vi "Read Dataset.vi"(8 "error in":errorcluster, 11 "Network Stream in":refnum<class "Network Stream.lvclass">) -> (0 "error out":errorcluster, 3 "Network Stream out":refnum<class "Network Stream.lvclass">)   [LabVIEW 2019, in "Network Stream.lvlib" / "Network Stream.lvclass"]
uses:
  Network Stream.lvclass
  C:/Program Files (x86)/National Instruments/LabVIEW 2019/vi.lib/ActorFramework/Actor/Actor.lvclass
  <vilib>/ActorFramework/Actor/Actor.lvclass/Actor.ctl
  Network Stream.lvclass/Network Stream.ctl
  Network Stream Messages/Dataset Msg/Dataset Msg.lvclass/Dataset Msg.ctl
  <vilib>/ActorFramework/Message Enqueuer/Message Enqueuer.lvclass/Message Enqueuer.ctl
  Network Stream Messages/NS Connection Msg/NS Connection Msg.lvclass/NS Connection Msg.ctl
  <vilib>/ActorFramework/Message Enqueuer/Enqueue.vi
  Network Stream Messages/Dataset Msg/Dataset Msg.lvclass
  C:/Program Files (x86)/National Instruments/LabVIEW 2019/vi.lib/ActorFramework/Message/Message.lvclass
  Network Stream Messages/NS Connection Msg/NS Connection Msg.lvclass
  <vilib>/ActorFramework/Message Priority Queue/Priority Enqueue.vi
  <resource>/objmgr/ni.dex.rc
  <vilib>/ActorFramework/Actor/Actor.lvclass
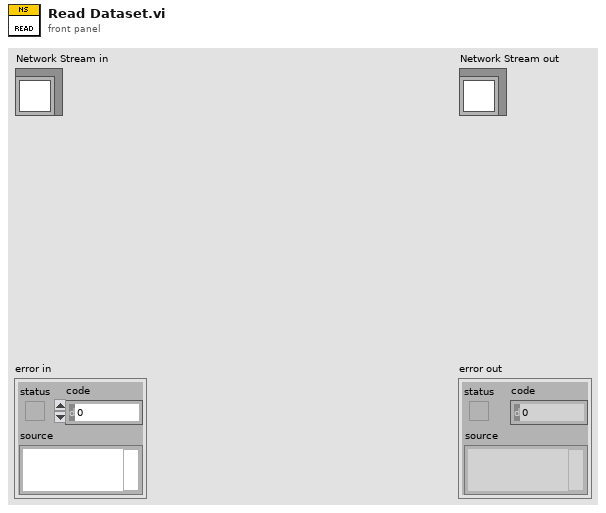
[diagram p1: front panel]
types:
  T1 = cluster{"System Status":cluster{"Power On Off":bool, "Discharge Temp":dbl, "Liquid Temp":dbl, "Suction Temp":dbl, "Ambient Temp":dbl, "Sleep":bool, "System Status":u16, "M1 Actuated":bool, "M2 Actuated":bool, "Sleep Timer":dbl, "M1 Bin":cluster{"Bin String":string, "Bin Color":u16}, "M2 Bin":cluster{"Bin String":string, "Bin Color":u16}, "Discharge Pressure":dbl, "Suction Pressure":dbl, "Compression Ratio":dbl, "Compressor Amps":dbl, "Compressor Hours":dbl, "Bypass Steps":u16, "SubCooling":dbl, "SuperHeat":dbl, "Serial Number":string, "EMO detected":bool, "EMO Tripped":bool, "Thermal cutoff":bool, "Thermal cutoff 2":bool, "High Pressure switch":bool, "Running Time":timestamp, "SOM Status":cluster{"Boot Up Time":timestamp, "Software Version":string, "CPU Usage":dbl, "Memory Available":dbl, "SD card free space":dbl, "SOM Storage":dbl}, "Cascade Extra":cluster{"Discharge Temp High Side":dbl, "Suction Temp High Side":dbl, "Liquid Temp High side":dbl, "Discharge Pressure 2":dbl, "Suction Pressure 2":dbl, "Low Side RPM":dbl, "High Side RPM":dbl}}, "M1 Status":cluster{"Case Temp":dbl, "Evap Temp":dbl, "Heater %":dbl, "EEV Steps":u32, "Set Temp":dbl, "Feedback":u8, "Power Drive":bool, "Piston Volts":dbl, "Safe Temp":bool, "Power":bool, "Thermal State":u16, "Error":bool, "In tollerance":bool, "Head State":u16, "Piston Force":dbl, "Package":string, "Dynamic SV":dbl, "PV":dbl, "TSD Temp":dbl, "DC Load Watts":dbl, "AC Load Watts":dbl, "Intec Feedback":dbl}, "M2 Status":cluster{"Case Temp":dbl, "Evap Temp":dbl, "Heater %":dbl, "EEV Steps":u32, "Set Temp":dbl, "Feedback":u8, "Power Drive":bool, "Piston Volts":dbl, "Safe Temp":bool, "Power":bool, "Thermal State":u16, "Error":bool, "In tollerance":bool, "Head State":u16, "Piston Force":dbl, "Package":string, "Dynamic SV":dbl, "PV":dbl, "TSD Temp":dbl, "DC Load Watts":dbl, "AC Load Watts":dbl, "Intec Feedback":dbl}, "Config Data":cluster{"Packages":cluster{"DUT Force lbf":cluster{" 0":u32, " 1":u32, " 2":u32, "3":u32, "4":u32, "5":u32, " 6":u32, "7":u32, "8":u32, "9":u32}, "DUT Names":cluster{"0":string, "1":string, "2":string, "3":string, "4":string, "5":string, "6":string, "7":string, "8":string, "9":string}}, "Heater PID":cluster{"P":dbl, "I":dbl, "D":dbl}, "Piston Settings":cluster{"Forces Slope":dbl, "Forces Intercept":dbl, "Transition Force":dbl, "Up Force":dbl, "Diameter (mm)":dbl, "Delay (ms)":dbl, "Pressure Ramp Delay (ms)":dbl}, "Safe Temps":cluster{"Minimum":i32, "Enabled":bool, "Maximum":i32}, "System Settings":cluster{"Number of Heads":i32, "60Hz Power":bool, "FTC200":bool, "AutoStartup":bool, "Purge":bool, "Sensors":bool, "HandClamp":bool, "ATE":bool, "Benchtop":bool, "Production":bool, "Refrigerant":u16, "Handler":bool, "Shuttle":bool, "220V":bool, "Cascade":bool, "Suction Sensor":u16, "Discharge Sensor":u16}, "Stepper Settings ":cluster{"Microstepping":u16, "Velocity":u8}, "Set Point Range":cluster{"Max":dbl, "Min":dbl}, "Pedestal Check DeltaT":dbl, "Ramp Delta T":dbl, "Ramp-SS Threshold":dbl, "SS Tolerance":dbl, "EEV PID":cluster{"Ramp Up Target":dbl, "Ramp Down Target":dbl, "Steady State Target":dbl, "Output":cluster{"Max":dbl, "Min":dbl}, "EBB and Flow Temp TH":dbl, "Cryomode EEV Max":dbl, "Valve minimum opening ":dbl, "Ramp Up EEV Steps":dbl, "Ramp Down EEV Steps":dbl, "SS EEV Steps Reset":dbl, "EBB and Flow Tol":dbl, "Gains":cluster{"P":dbl, "I":dbl, "D":dbl}, "Dissabled Target":dbl, "CryoMode Gains":cluster{"P":dbl, "I":dbl, "D":dbl}, "M1 SuperHeat Setpoint":dbl, "M2 Gains":cluster{"P":dbl, "I":dbl, "D":dbl}, "Flow Curve":u16}, "Sleep Timeout":dbl, "Bypass Values":cluster{"Bypass Valve":bool, "Flow Curve":u16, "Output":cluster{"Max":u32, "Min":u32}, "Feedback":u16, "Cyth Bypass":bool, "PID":cluster{"P":dbl, "I":dbl, "D":dbl}, "Pressure setpoint":i16, "Cryo Temp":i16, "Superheat Setpoint":i16, "Cryo Setpoint":i16}, "Default Temp":dbl, "InTEC":cluster{"Enabled":bool, "IP":string, "Port":u16}, "M1 TSD":cluster{"Gain":dbl, "Offset":dbl, "V Offset ":dbl}, "M2 TSD":cluster{"Gain":dbl, "Offset":dbl, "V Offset ":dbl}, "M1 T-Case Calibration":cluster{"Gain":dbl, "Offset":dbl}, "M2 T-Case Calibration":cluster{"Gain":dbl, "Offset":dbl}, "Heater PID TSD":cluster{"P":dbl, "I":dbl, "D":dbl}, "M2 Heater PID":cluster{"P":dbl, "I":dbl, "D":dbl}}}
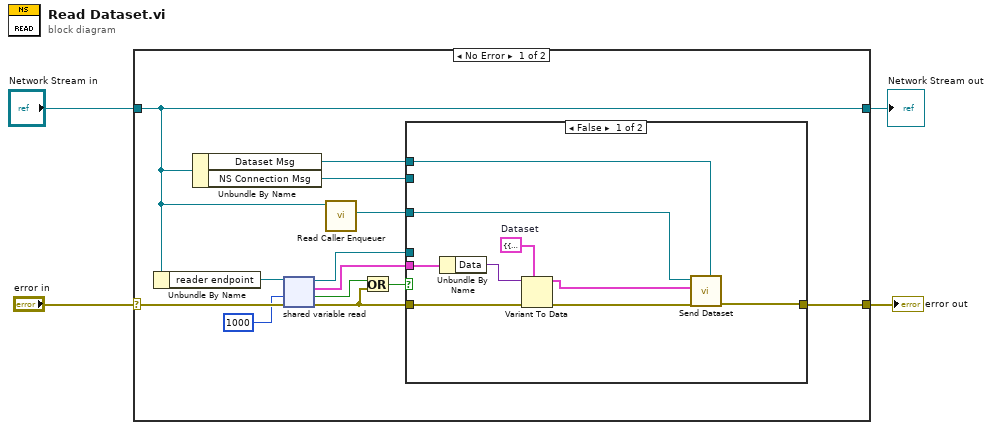
[diagram p0: block diagram]
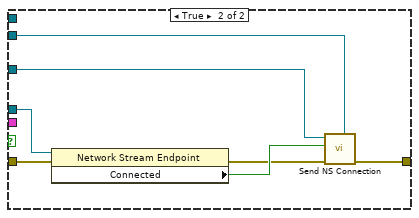
[diagram p2: hidden frame]
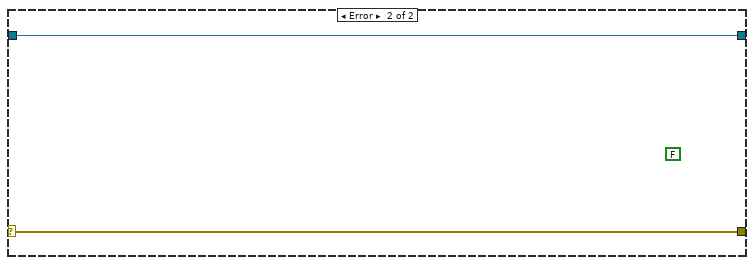
[diagram p3: hidden frame]
diagram:
  n1 = case shown="No Error" "error in" {
    selector: "error in" -> [w17 w35]
    tunnel: [w14 w35] -> w3
    tunnel: [w7 w34] -> w1
    tunnel: "Network Stream in" -> [w7 w34]
    frame No Error {
      n2 = Unbundle By Name(w7) -> ("reader endpoint"=w13:refnum<k21>)
      n3 = Unbundle By Name(w7) -> ("Dataset Msg"=w5:refnum<class "Dataset Msg.lvclass">, "NS Connection Msg"=w11:refnum<class "NS Connection Msg.lvclass">)
      n4 = shared-variable-read(w13, w17, 1000 ("timeout ms (-1)")) -> (w12:refnum<k21>, w8:errorcluster, w10:bool, w15:cluster{"Data":variant, "Timestamp":timestamp})
      n5 = call <vilib>:"Read Caller Enqueuer.vi"("Actor"=w7) -> ("Caller Enqueuer"=w6:refnum<class "Message Enqueuer.lvclass">)  [unwired: 10 in]
      n6 = Or(x=w10, y=w8) -> (x .or. y?=w9:bool)
      n7 = case shown="False" w9 {
        tunnel: w8 -> [w25 w31]
        tunnel: w15 -> [w24 _]
        tunnel: [w22 w28] -> w14
        tunnel: w12 -> [_ w33]
        tunnel: w11 -> [_ w30]
        tunnel: w6 -> [w21 w27]
        tunnel: w5 -> [w20 _]
        frame False {
          w18 = T1 {"System Status"={"Power On Off"=FALSE, "Discharge Temp"=0.0, "Liquid Temp"=0.0, "Suction Temp"=0.0, "Ambient Temp"=0.0, "Sleep"=FALSE, "System Status"=0, "M1 Actuated"=FALSE, "M2 Actuated"=FALSE, "Sleep Timer"=0.0, "M1 Bin"={"Bin String"="", "Bin Color"=1}, "M2 Bin"={"Bin String"="", "Bin Color"=1}, "Discharge Pressure"=0.0, "Suction Pressure"=0.0, "Compression Ratio"=0.0, "Compressor Amps"=0.0, "Compressor Hours"=0.0, "Bypass Steps"=0, "SubCooling"=0.0, "SuperHeat"=0.0, "Serial Number"="", "EMO detected"=FALSE, "EMO Tripped"=FALSE, "Thermal cutoff"=FALSE, "Thermal cutoff 2"=FALSE, "High Pressure switch"=FALSE, "Running Time"=timestamp(0 s since 1904-01-01), "SOM Status"={"Boot Up Time"=timestamp(0 s since 1904-01-01), "Software Version"="", "CPU Usage"=0.0, "Memory Available"=0.0, "SD card free space"=0.0, "SOM Storage"=0.0}, "Cascade Extra"={"Discharge Temp High Side"=0.0, "Suction Temp High Side"=0.0, "Liquid Temp High side"=0.0, "Discharge Pressure 2"=0.0, "Suction Pressure 2"=0.0, "Low Side RPM"=0.0, "High Side RPM"=0.0}}, "M1 Status"={"Case Temp"=0.0, "Evap Temp"=0.0, "Heater %"=0.0, "EEV Steps"=0, "Set Temp"=0.0, "Feedback"=0, "Power Drive"=FALSE, "Piston Volts"=0.0, "Safe Temp"=FALSE, "Power"=FALSE, "Thermal State"=0, "Error"=FALSE, "In tollerance"=FALSE, "Head State"=0, "Piston Force"=0.0, "Package"="", "Dynamic SV"=0.0, "PV"=0.0, "TSD Temp"=0.0, "DC Load Watts"=0.0, "AC Load Watts"=0.0, "Intec Feedback"=0.0}, "M2 Status"={"Case Temp"=0.0, "Evap Temp"=0.0, "Heater %"=0.0, "EEV Steps"=0, "Set Temp"=0.0, "Feedback"=0, "Power Drive"=FALSE, "Piston Volts"=0.0, "Safe Temp"=FALSE, "Power"=FALSE, "Thermal State"=0, "Error"=FALSE, "In tollerance"=FALSE, "Head State"=0, "Piston Force"=0.0, "Package"="", "Dynamic SV"=0.0, "PV"=0.0, "TSD Temp"=0.0, "DC Load Watts"=0.0, "AC Load Watts"=0.0, "Intec Feedback"=0.0}, "Config Data"={"Packages"={"DUT Force lbf"={" 0"=0, " 1"=0, " 2"=0, "3"=0, "4"=0, "5"=0, " 6"=0, "7"=0, "8"=0, "9"=0}, "DUT Names"={"0"="", "1"="", "2"="", "3"="", "4"="", "5"="", "6"="", "7"="", "8"="", "9"=""}}, "Heater PID"={"P"=0.0, "I"=0.0, "D"=0.0}, "Piston Settings"={"Forces Slope"=0.0, "Forces Intercept"=0.0, "Transition Force"=0.0, "Up Force"=0.0, "Diameter (mm)"=0.0, "Delay (ms)"=0.0, "Pressure Ramp Delay (ms)"=0.0}, "Safe Temps"={"Minimum"=17, "Enabled"=TRUE, "Maximum"=95}, "System Settings"={"Number of Heads"=0, "60Hz Power"=TRUE, "FTC200"=TRUE, "AutoStartup"=FALSE, "Purge"=TRUE, "Sensors"=TRUE, "HandClamp"=TRUE, "ATE"=TRUE, "Benchtop"=TRUE, "Production"=TRUE, "Refrigerant"=0, "Handler"=TRUE, "Shuttle"=TRUE, "220V"=FALSE, "Cascade"=FALSE, "Suction Sensor"=0, "Discharge Sensor"=0}, "Stepper Settings "={"Microstepping"=0, "Velocity"=8}, "Set Point Range"={"Max"=0.0, "Min"=0.0}, "Pedestal Check DeltaT"=0.0, "Ramp Delta T"=0.0, "Ramp-SS Threshold"=0.0, "SS Tolerance"=0.0, "EEV PID"={"Ramp Up Target"=0.0, "Ramp Down Target"=0.0, "Steady State Target"=0.0, "Output"={"Max"=0.0, "Min"=0.0}, "EBB and Flow Temp TH"=0.0, "Cryomode EEV Max"=0.0, "Valve minimum opening "=0.0, "Ramp Up EEV Steps"=0.0, "Ramp Down EEV Steps"=0.0, "SS EEV Steps Reset"=0.0, "EBB and Flow Tol"=0.0, "Gains"={"P"=0.0, "I"=0.0, "D"=0.0}, "Dissabled Target"=0.0, "CryoMode Gains"={"P"=0.0, "I"=0.0, "D"=0.0}, "M1 SuperHeat Setpoint"=0.0, "M2 Gains"={"P"=0.0, "I"=0.0, "D"=0.0}, "Flow Curve"=0}, "Sleep Timeout"=0.0, "Bypass Values"={"Bypass Valve"=TRUE, "Flow Curve"=0, "Output"={"Max"=0, "Min"=0}, "Feedback"=0, "Cyth Bypass"=TRUE, "PID"={"P"=0.0, "I"=0.0, "D"=0.0}, "Pressure setpoint"=0, "Cryo Temp"=0, "Superheat Setpoint"=0, "Cryo Setpoint"=0}, "Default Temp"=0.0, "InTEC"={"Enabled"=FALSE, "IP"="192.168.1.100", "Port"=5000}, "M1 TSD"={"Gain"=0.0, "Offset"=0.0, "V Offset "=0.0}, "M2 TSD"={"Gain"=0.0, "Offset"=0.0, "V Offset "=0.0}, "M1 T-Case Calibration"={"Gain"=0.0, "Offset"=0.0}, "M2 T-Case Calibration"={"Gain"=0.0, "Offset"=0.0}, "Heater PID TSD"={"P"=0.0, "I"=0.0, "D"=0.0}, "M2 Heater PID"={"P"=0.0, "I"=0.0, "D"=0.0}}}  # Dataset
          n8 = Unbundle By Name(w24) -> ("Data"=w26:variant)
          n9 = Variant To Data(error in=w25, type=w18, Variant=w26) -> (data=w19:T1, error out=w23:errorcluster)
          n10 = call "Send Dataset.vi"("Message Type"=w20, "error in (no error)"=w23, "Dataset"=w19, "Message Enqueuer"=w21) -> ("error out"=w22:errorcluster)  [unwired: 6 in, 1 out]
        }
        frame True {
          n11 = property class="Network Stream Endpoint"(reference=w33, error in=w31) -> (error out=w29:errorcluster, "Connected"=w32:bool)  [unwired: 1 out]
          n12 = call "Send NS Connection.vi"("Message Type"=w30, "error in (no error)"=w29, "NS Conn"=w32, "Message Enqueuer"=w27) -> ("error out"=w28:errorcluster)  [unwired: 6 in, 1 out]
        }
      }
    }
    frame Error {
      (unwired) FALSE ("Connected")
    }
  }
  "error out" <- w3
  "Network Stream out" <- w1
